vi "Write TSP.vi"(8 "error in (no error)":errorcluster, 10 "TSP":sgl, 11 "TE Cooler in":refnum<class "TE Cooler.lvclass">) -> (0 "error out":errorcluster, 3 "TE Cooler out":refnum<class "TE Cooler.lvclass">)   [LabVIEW 2014, in "TE Cooler.lvlib" / "TE Cooler.lvclass"]
uses:
  TE Cooler.lvclass
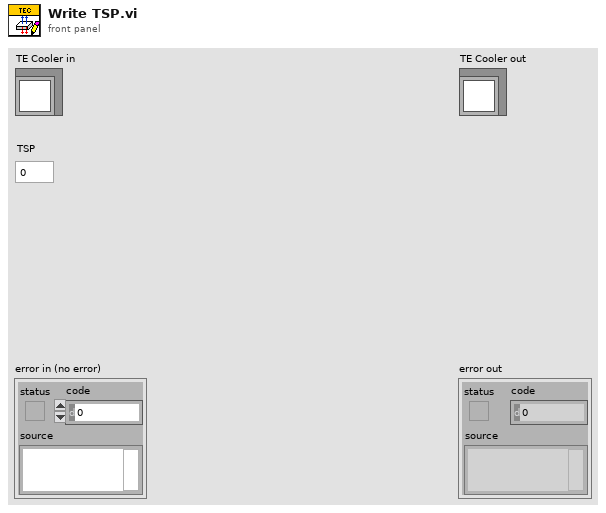
[diagram p1: front panel]
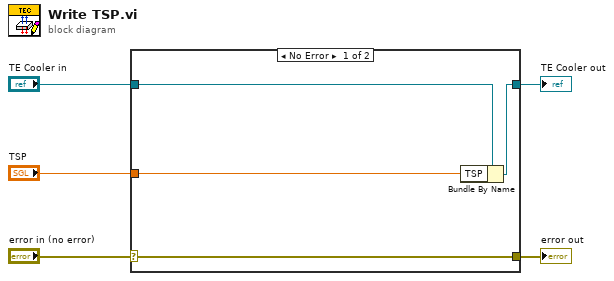
[diagram p0: block diagram]
diagram:
  n1 = case shown="No Error" "error in (no error)" {
    selector: "error in (no error)" -> [w9 w10]
    tunnel: [w9 w10] -> w4
    tunnel: [w7 w11] -> w2
    tunnel: "TE Cooler in" -> [w8 w11]
    tunnel: "TSP" -> [w6 _]
    frame No Error {
      n2 = Bundle By Name(cluster=w8, "TSP"=w6) -> (w7:refnum<class "TE Cooler.lvclass">)
    }
    frame Error {
    }
  }
  "error out" <- w4
  "TE Cooler out" <- w2
